vi "LJM logger startup config check.vi"(8 "Good Config?":bool, 10 "Config Name":string="config.cfg", 11 "Config Error In":errorcluster) -> (2 "Force Defaults":bool)   [LabVIEW 2026]
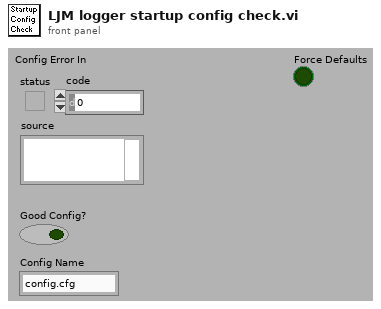
[diagram p1: front panel]
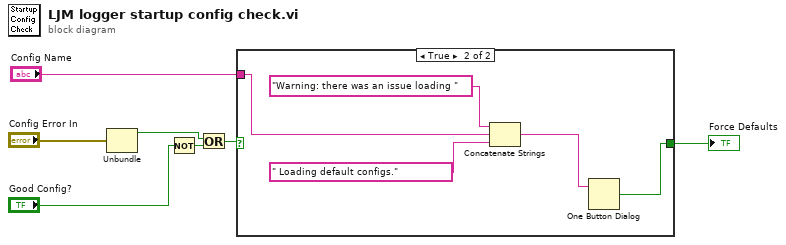
[diagram p0: block diagram]
diagram:
  n1 = Unbundle("Config Error In") -> ("status"=w4:bool)  [unwired: 2 out]
  n2 = Not(x="Good Config?") -> (.not. x?=w6:bool)
  n3 = Or(x=w4, y=w6) -> (x .or. y?=w3:bool)
  n4 = case shown="True" w3 {
    selector: w3 -> [w8 _]
    tunnel: [w8 w13] -> w2
    tunnel: "Config Name" -> [_ w10]
    frame False {
    }
    frame True {
      n5 = Concatenate Strings("Warning: there was an issue loading " ("message"), w10, " Loading default configs." ("message")) -> (w9:string)
      n6 = One Button Dialog(message=w9) -> (true=w13:bool)  [unwired: 1 in]
    }
  }
  "Force Defaults" <- w2
